vi "Get String Contol Reference.vi"(11 "error in (no error)":errorcluster) -> (4 "String":refnum<vi>, 6 "vi reference":refnum<vi>, 15 "error out":errorcluster)   [LabVIEW 2021, in "Migrator.lvlib"]
uses:
  Migrator.lvlib
  Path Functions/Path Functions.lvlib
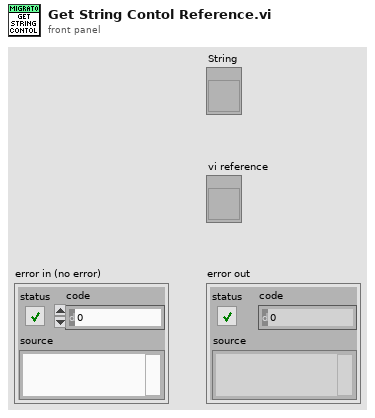
[diagram p1: front panel]
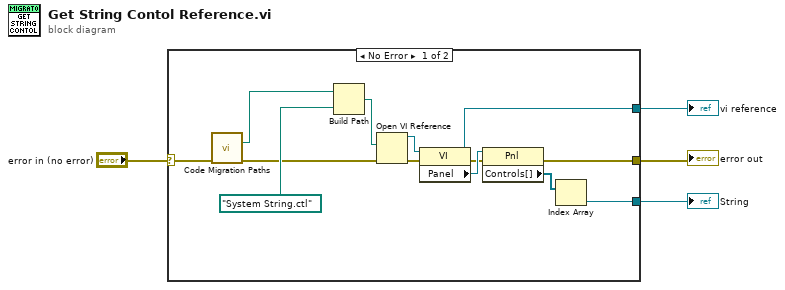
[diagram p0: block diagram]
diagram:
  n1 = case shown="No Error" "error in (no error)" {
    selector: "error in (no error)" -> [w7 w18]
    tunnel: [w8 _] -> w4
    tunnel: [w6 w18] -> w2
    tunnel: [w5 _] -> w1
    frame No Error {
      n2 = call "Code Migration Paths.vi"("error in (no error)"=w7) -> ("IO Controls"=w16:path, "error out"=w12:errorcluster)  [unwired: 6 in, 7 out]
      n3 = Build Path(base path=w16, name or relative path=path "System String.ctl") -> (appended path=w15:path)
      n4 = Open VI Reference(vi path=w15, error in (no error)=w12) -> (vi reference=w9:refnum<vi>, error out=w11:errorcluster)  [unwired: 4 in]
      n5 = property class="VI"(reference=w9, error in=w11) -> (reference out=w5:refnum<vi>, error out=w10:errorcluster, "Panel"=w14:refnum<vi>)
      n6 = property class="Pnl"(reference=w14, error in=w10) -> (error out=w6:errorcluster, "Controls[]"=w13:refnum<vi>[])  [unwired: 1 out]
      n7 = Index Array(array=w13) -> (element=w8:refnum<vi>)  [unwired: 1 in]
    }
    frame Error {
    }
  }
  "String" <- w4
  "error out" <- w2
  "vi reference" <- w1
